vi "stop.vi"(3 "error in (no error)":errorcluster, 4 "stop":bool, 5 "K2602 in":refnum<class "K2602.lvclass">) -> (0 "error out":errorcluster, 1 "Stopped":bool, 2 "K2602 out":refnum<class "K2602.lvclass">)   [LabVIEW 2011, in "Hardware.lvlib" / "Channels.lvlib" / "K2602.lvclass"]
doc: "Abstract Method.\n\nStops the analog output. This vi indicates of the analog output has stopped, and can be used to actively stop the output."
uses:
  K2602.lvclass
  K2602.lvclass/K2602.ctl
  <instrlib>/Keithley 2600 Series/Keithley 2600 Series.lvlib
panel:
  out "Boolean array":bool[](array[boolean])
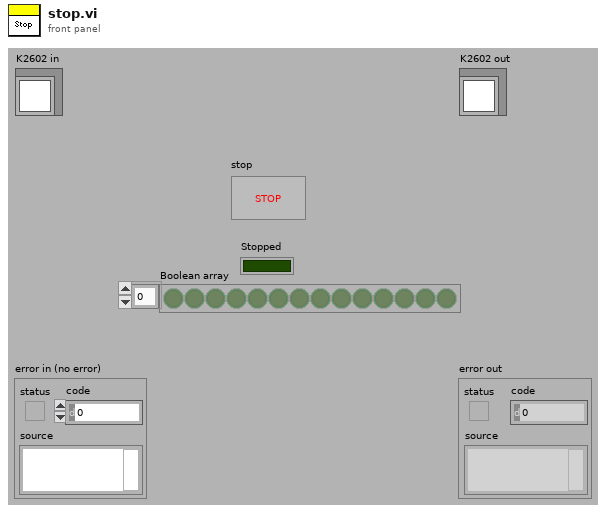
[diagram p1: front panel]
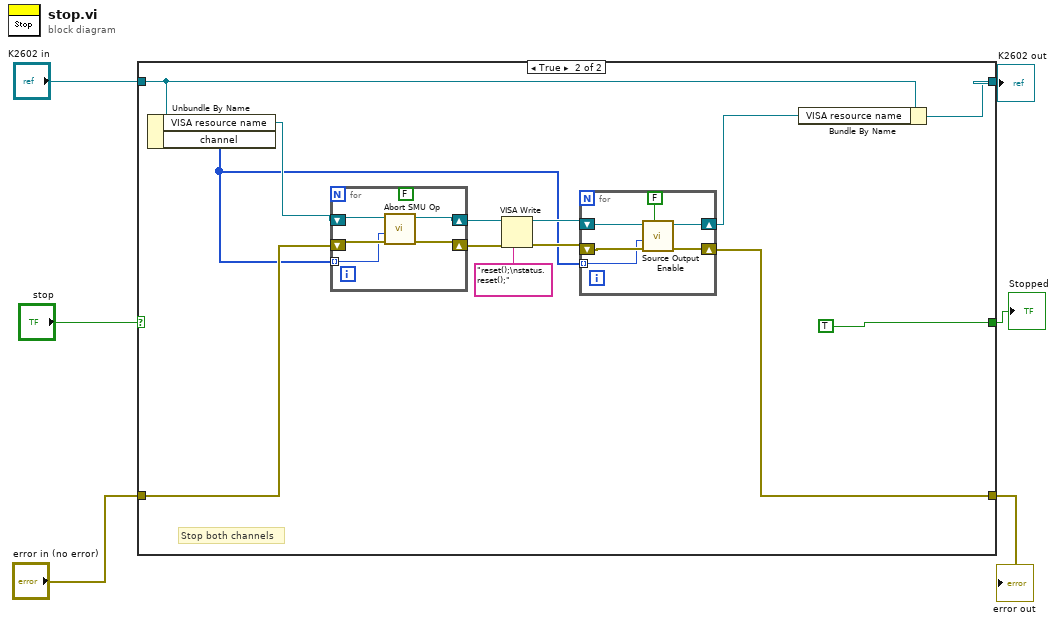
[diagram p0: block diagram]
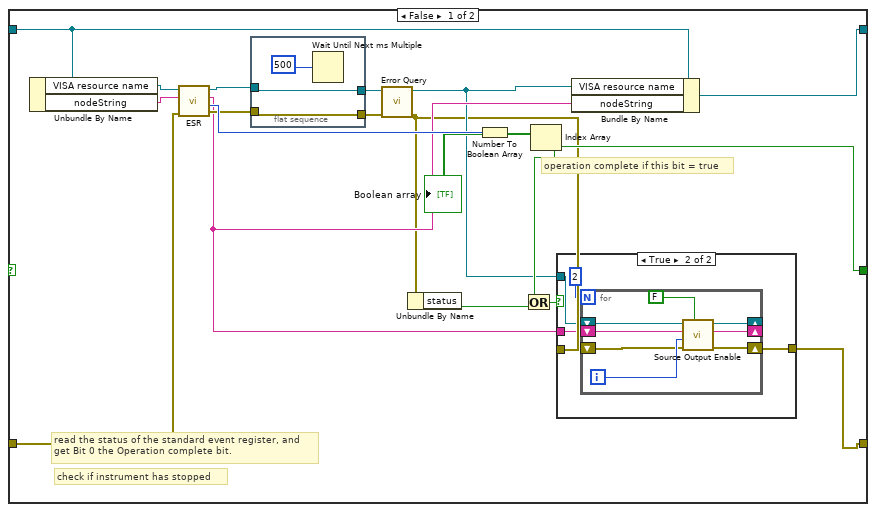
[diagram p2: hidden frame]
diagram:
  n1 = case shown="True" "stop" {
    tunnel: "error in (no error)" -> [w23 w46]
    tunnel: [w16 w44] -> w2
    tunnel: [w15 TRUE] -> w1
    tunnel: [w21 w53] -> w5
    tunnel: "K2602 in" -> [w20 w54]
    frame False {
      # "operation complete if this bit = true"
      # "read the status of the standard event register, and \nget Bit 0 the Operation complete bit."
      # "check if instrument has stopped"
      n2 = Unbundle By Name(w20) -> ("VISA resource name"=w14:refnum<visa-resource-name>, "nodeString"=w24:string)
      n3 = call <instrlib>:"ESR.vi"("error in (no error)"=w23, "Node In"=w24, "VISA resource name"=w14) -> ("error out"=w18:errorcluster, "ESR"=w22:u8, "Node Out"=w13:string, "VISA resource name out"=w17:refnum<visa-resource-name>)  [unwired: 4 in, 1 out]
      n4 = flat-sequence {
        tunnel: w18 -> [w25]
        tunnel: w17 -> [w26]
        tunnel: [w25] -> w11
        tunnel: [w26] -> w12
        frame #0 {
          n5 = Wait Until Next ms Multiple(millisecond multiple=500) -> ()  [unwired: 1 out]
        }
      }
      n6 = call <instrlib>:"Error Query.vi"("error in (no error)"=w11, "VISA resource name"=w12) -> ("error out"=w9:errorcluster, "VISA resource name out"=w10:refnum<visa-resource-name>)  [unwired: 6 in, 2 out]
      n7 = Unbundle By Name(w9) -> ("status"=w8:bool)
      n8 = Number To Boolean Array(number=w22) -> (Boolean array=w19:bool[])
      "Boolean array" <- w19
      n9 = Index Array(array=w19) -> (element=w15:bool)  [unwired: 1 in]
      n10 = Or(x=w15, y=w8) -> (x .or. y?=w7:bool)
      n11 = case shown="True" w7 {
        tunnel: w9 -> [w28 w33]
        tunnel: [w28 w32] -> w16
        tunnel: w10 -> [_ w31]
        tunnel: w13 -> [_ w30]
        frame False {
        }
        frame True {
          n12 = for {
            N: 2 -> [_]
            shift-right: [w39] -> _
            shift-left: w31 -> [w36]
            shift-right: [w38] -> _
            shift-left: w30 -> [w35]
            shift-right: [w37] -> w32
            shift-left: w33 -> [w34]
            i -> [w41]
            n13 = call <instrlib>:"Source Output Enable.vi"("Output (Off)"=FALSE, "error in (no error)"=w34, "Channel (Channel A)"=w41, "Node In"=w35, "VISA resource name"=w36) -> ("error out"=w37:errorcluster, "Node Out"=w38:string, "VISA resource name out"=w39:refnum<visa-resource-name>)  [unwired: 3 in, 1 out]
          }
        }
      }
      n14 = Bundle By Name(cluster=w20, "VISA resource name"=w10, "nodeString"=w13) -> (w21:refnum<class "K2602.lvclass">)
    }
    frame True {
      # "Stop both channels"
      n15 = Unbundle By Name(w54) -> ("VISA resource name"=w47:refnum<visa-resource-name>, "channel"=w42:i32[])
      n16 = for {
        shift-right: [w62] -> w50
        shift-left: w47 -> [w65]
        shift-right: [w61] -> w49
        shift-left: w46 -> [w64]
        tunnel: w42 -> [w63] mode=indexing
        (unwired) FALSE ("Output (Off)")
        n17 = call <instrlib>:"Abort SMU Op.vi"("error in"=w64, "Channel (Channel A)"=w63, "VISA resource name"=w65) -> ("error out"=w61:errorcluster, "VISA resource name out"=w62:refnum<visa-resource-name>)  [unwired: 5 in, 2 out]
      }
      n18 = VISA Write(VISA resource name=w50, write buffer="reset();\nstatus.reset();", error in (no error)=w49) -> (VISA resource name out=w48:refnum<visa-resource-name>, error out=w45:errorcluster)  [unwired: 1 out]
      n19 = for {
        shift-right: [w59] -> w43
        shift-left: w48 -> [w57]
        shift-right: [w58] -> w44
        shift-left: w45 -> [w56]
        tunnel: w42 -> [w55] mode=indexing
        n20 = call <instrlib>:"Source Output Enable.vi"("Output (Off)"=FALSE, "error in (no error)"=w56, "Channel (Channel A)"=w55, "VISA resource name"=w57) -> ("error out"=w58:errorcluster, "VISA resource name out"=w59:refnum<visa-resource-name>)  [unwired: 4 in, 2 out]
      }
      n21 = Bundle By Name(cluster=w54, "VISA resource name"=w43) -> (w53:refnum<class "K2602.lvclass">)
    }
  }
  "error out" <- w2
  "K2602 out" <- w5
  "Stopped" <- w1
